vi "DecodeVireoToBotSpeak.vi"(3 "Via file":string="// Autogenerated Vireo assembly file\n// Generated on Fri Mar 27 10:48:11 2015\n\ndefine (c0 dv(.UInt32 1) )\ndefine (c1 dv(.UInt32 1) )\ndefine (c2 dv(c(\n    e(.String n0)   // Address\n    e(.String n1)   // Reply EOF\n    e(.String n2)   // Hardware\n    e(.Int8 n3)   // Retries\n    e(.Int32 n4)   // Timeout\n    e(.Boolean n5)   // Open?\n) ('' '' '' 0 0 false )) )\ndefine (c3 dv(.String '') )\n//---------------------------------------------------\n//VI Definition: BotSpeak_DIOWrite.vi\ndefine (videf1 dv(.VirtualInstrument (\n    c(\n        i(dv(.UInt32 1) local2)   // State\n        o(dv(.String '') local5)   // response\n        i(dv(c(\n            e(.String n0)   // Address\n            e(.String n1)   // Reply EOF\n            e(.String n2)   // Hardware\n            e(.Int8 n3)   // Retries\n            e(.Int32 n4)   // Timeout\n            e(.Boolean n5)   // Open?\n        ) ('' '' '' 0 0 false )) local1)   // Bot Settings\n        i(dv(.UInt32 0) local3)   // DIO Line\n        o(dv(c(\n            e(.String n0)   // Address\n            e(.String n1)   // Reply EOF\n            e(.String n2)   // Hardware\n            e(.Int8 n3)   // Retries\n            e(.Int32 n4)   // Timeout\n            e(.Boolean n5)   // Open?\n        ) ('' '' '' 0 0 false )) local4)   // Bot Settings\n    )\n    c(\n    )\n        clump(1\n        Copy(c2 local4 )\n        Copy(c3 local5 )\n//--- end of vi\n    )\n)))\n//---------------------------------------------------\n//VI Definition: TestingVI.vi\ndefine (videf2 dv(.VirtualInstrument (\n    c(\n    )\n        clump(1\n        videf1(c0 * * c1 *)\n//--- end of vi\n    )\n)))\nenqueue (videf2)\n") -> (1 "BotSpeak":string="SET DIO[1],1\n")   [LabVIEW 2014]
panel:
  out "Array 3":string[](array[string])=["", "", "", "", "BotSpeak_DIOWrite.vi", "TestingVI.vi", ""]
  out "Params":cluster{"Constant":string, "value":string}[](array[cluster])=[{"Constant"="videf1", "value"="SET DIO[#],#: 3 0 \n"}, {"Constant"="c3", "value"="''"}, {"Constant"="c2", "value"="   e(.String n0)   // Address\n    e(.String n1)   // Reply EOF\n    e(.String n2)   // Hardware\n    e(.Int8 n3)   // Retries\n    e(.Int32 n4)   // Timeout\n    e(.Boolean n5)   // Open?\n) ('' '' '' 0 0 false )"}, {"Constant"="c1", "value"="1"}, {"Constant"="c0", "value"="1"}]
  out "Array":T1(array[cluster])=[{"command"="define", "Contents"="c0 dv(.UInt32 1)", "previous comment"="// Generated on Fri Mar 27 10:48:11 2015"}, {"command"="define", "Contents"="c1 dv(.UInt32 1)", "previous comment"=""}, {"command"="define", "Contents"="c2 dv(c(\n    e(.String n0)   // Address\n    e(.String n1)   // Reply EOF\n    e(.String n2)   // Hardware\n    e(.Int8 n3)   // Retries\n    e(.Int32 n4)   // Timeout\n    e(.Boolean n5)   // Open?\n) ('' '' '' 0 0 false ))", "previous comment"=""}, {"command"="define", "Contents"="c3 dv(.String '')", "previous comment"=""}, {"command"="define", "Contents"="videf1 dv(.VirtualInstrument (\n    c(\n        i(dv(.UInt32 1) local2)   // State\n        o(dv(.String '') local5)   // response\n        i(dv(c(\n            e(.String n0)   // Address\n            e(.String n1)   // Reply EOF\n            e(.String n2)   // Hardware\n            e(.Int8 n3)   // Retries\n            e(.Int32 n4)   // Timeout\n            e(.Boolean n5)   // Open?\n        ) ('' '' '' 0 0 false )) local1)   // Bot Settings\n        i(dv(.UInt32 0) local3)   // DIO Line\n        o(dv(c(\n            e(.String n0)   // Address\n            e(.String n1)   // Reply EOF\n            e(.String n2)   // Hardware\n            e(.Int8 n3)   // Retries\n            e(.Int32 n4)   // Timeout\n            e(.Boolean n5)   // Open?\n        ) ('' '' '' 0 0 false )) local4)   // Bot Settings\n    )\n    c(\n    )\n        clump(1\n        Copy(c2 local4 )\n        Copy(c3 local5 )\n//--- end of vi\n    )\n))", "previous comment"="//VI Definition: BotSpeak_DIOWrite.vi"}, {"command"="define", "Contents"="videf2 dv(.VirtualInstrument (\n    c(\n    )\n        clump(1\n        videf1(c0 * * c1 *)\n//--- end of vi\n    )\n))", "previous comment"="//VI Definition: TestingVI.vi"}, {"command"="enqueue", "Contents"="videf2", "previous comment"=""}]
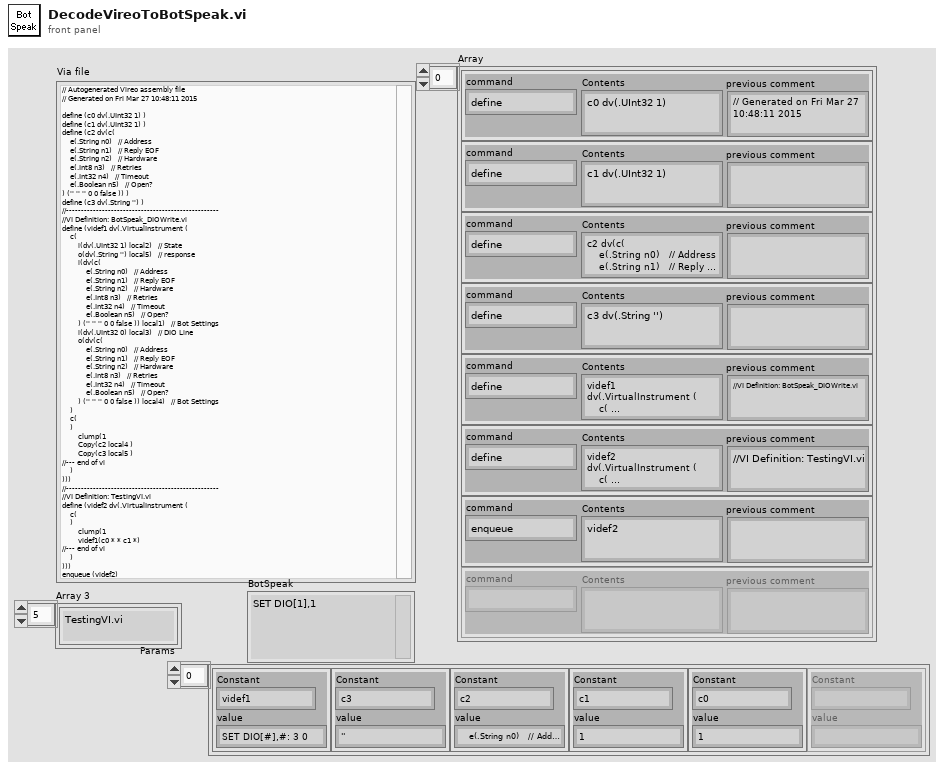
[diagram p1: front panel]
types:
  T1 = cluster{"command":string, "Contents":string, "previous comment":string}[]
  T2 = cluster{"Contents":string, "Contents 2":string}[]
  T3 = cluster{"command":string, "Contents":string, "Via file":string}
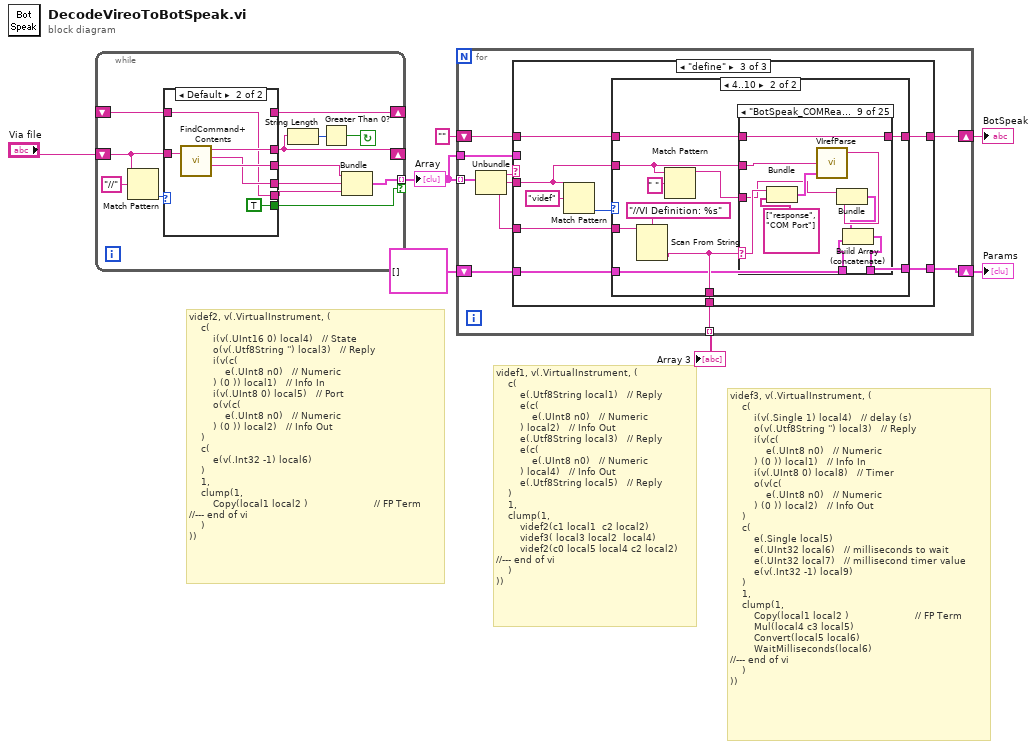
[diagram p0: block diagram]
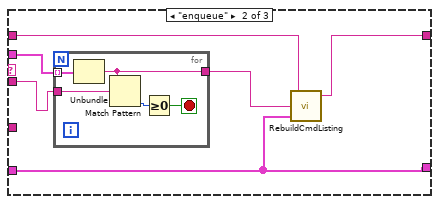
[diagram p3: hidden frame]
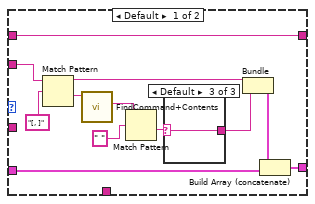
[diagram p4: hidden frame]
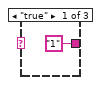
[diagram p5: hidden frame]
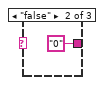
[diagram p6: hidden frame]
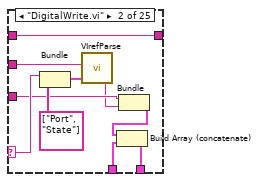
[diagram p8: hidden frame]
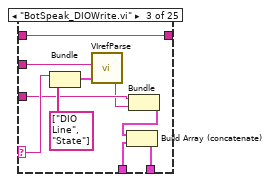
[diagram p9: hidden frame]
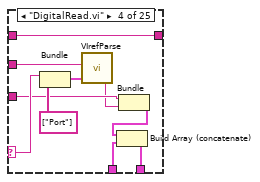
[diagram p10: hidden frame]
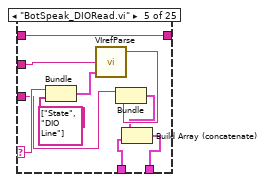
[diagram p11: hidden frame]
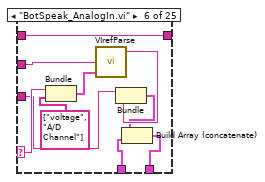
[diagram p12: hidden frame]
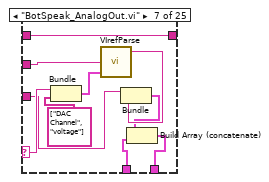
[diagram p13: hidden frame]
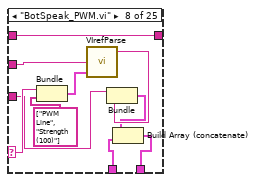
[diagram p14: hidden frame]
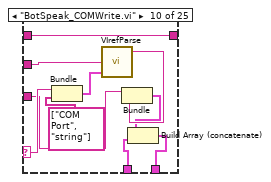
[diagram p15: hidden frame]
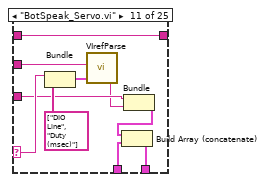
[diagram p16: hidden frame]
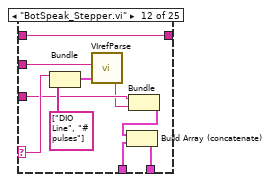
[diagram p17: hidden frame]
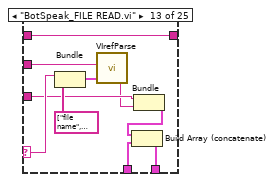
[diagram p18: hidden frame]
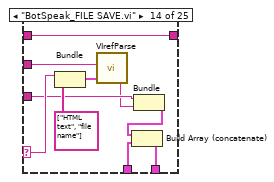
[diagram p19: hidden frame]
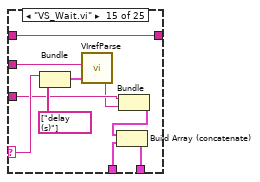
[diagram p20: hidden frame]
diagram:
  # "videf3, v(.VirtualInstrument, (\n    c(\n        i(v(.Single 1) local4)   // delay (s)\n        o(v(.Utf8String '') local3)   // Reply\n        i(v(c(\n            e(.UInt8 n0)   // Numeric\n        ) (0 )) local1)   // Info In\n        i(v(.UInt8 0) local8)   // Timer\n        o(v(c(\n            e(.UInt8 n0)   // Numeric\n        ) (0 )) local2)   // Info Out\n    )\n    c(\n        e(.Single local5)\n        e(.UInt32 local6)   // milliseconds to wait\n        e(.UInt32 local7)   // millisecond timer value\n        e(v(.Int32 -1) local9)\n    )\n    1,\n    clump(1,\n        Copy(local1 local2 )                      // FP Term\n        Mul(local4 c3 local5)\n        Convert(local5 local6)\n        WaitMilliseconds(local6)\n//--- end of vi\n    )\n))"
  # "videf1, v(.VirtualInstrument, (\n    c(\n        e(.Utf8String local1)   // Reply\n        e(c(\n            e(.UInt8 n0)   // Numeric\n        ) local2)   // Info Out\n        e(.Utf8String local3)   // Reply\n        e(c(\n            e(.UInt8 n0)   // Numeric\n        ) local4)   // Info Out\n        e(.Utf8String local5)   // Reply\n    )\n    1,\n    clump(1,\n        videf2(c1 local1  c2 local2)\n        videf3( local3 local2  local4)\n        videf2(c0 local5 local4 c2 local2)\n//--- end of vi\n    )\n))"
  # "videf2, v(.VirtualInstrument, (\n    c(\n        i(v(.UInt16 0) local4)   // State\n        o(v(.Utf8String '') local3)   // Reply\n        i(v(c(\n            e(.UInt8 n0)   // Numeric\n        ) (0 )) local1)   // Info In\n        i(v(.UInt8 0) local5)   // Port\n        o(v(c(\n            e(.UInt8 n0)   // Numeric\n        ) (0 )) local2)   // Info Out\n    )\n    c(\n        e(v(.Int32 -1) local6)\n    )\n    1,\n    clump(1,\n        Copy(local1 local2 )                      // FP Term\n//--- end of vi\n    )\n))"
  n1 = while {
    shift-right: [w20] -> _
    shift-left: "Via file" -> [w14]
    tunnel: [w15] -> w1 mode=indexing if=w9
    shift-right: [w11] -> _
    shift-left: _ -> [w10]
    stop <- w18 continue-if-true
    n2 = Match Pattern(string=w14, regular expression="//") -> (offset past match=w12:i32)  [unwired: 1 in, 3 out]
    n3 = case shown="Default" w12 {
      tunnel: [w23 w31] -> w20
      tunnel: ["//" ("regular expression") w30] -> w17
      tunnel: [w21 w29] -> w16
      tunnel: w14 -> [w25 w28]
      tunnel: [w21 _] -> w11
      tunnel: [_ w27] -> w8
      tunnel: w10 -> [_ w27]
      tunnel: [_ TRUE] -> w9
      frame 0..2 {
        n4 = Match Pattern(string=w25, regular expression="\n") -> (before substring=w21:string, after substring=w23:string)  [unwired: 1 in, 2 out]
      }
      frame Default {
        n5 = call <vilib>:"FindCommand+Contents.vi"("Via file in"=w28) -> ("left"=w31:string, "Contents"=w29:string, "command"=w30:string)  [unwired: 1 in, 1 out]
      }
    }
    n6 = String Length(string=w20) -> (length=w19:i32)
    n7 = Greater Than 0?(x=w19) -> (x > 0?=w18:bool)
    n8 = Bundle("command"=w17, "Contents"=w16, "Via file"=w8) -> (w15:T3)  [unwired: 1 in]
  }
  "Array" <- w1
  n9 = for {
    tunnel: w1 -> [w41] mode=indexing
    shift-right: [w36] -> w5
    shift-left: "" -> [w37]
    shift-right: [w35] -> w3
    shift-left: T2 [] -> [w34]
    tunnel: [w33] -> w2 mode=indexing
    tunnel: w1 -> [w32]
    n10 = Unbundle(w41) -> ("command"=w40:string, "Contents"=w39:string, "Via file"=w38:string)
    n11 = case shown="\"define\"" w40 {
      tunnel: w39 -> [_ w46 w58]
      tunnel: w38 -> [_ _ w61]
      tunnel: w37 -> [w42 w48 w60]
      tunnel: [w42 w49 w59] -> w36
      tunnel: [w43 w44 w57] -> w35
      tunnel: w34 -> [w43 w44 w56]
      tunnel: [_ _ w55] -> w33
      tunnel: w32 -> [_ w47 _]
      frame Default {
      }
      frame "enqueue" {
        n12 = for {
          tunnel: w47 -> [w54] mode=indexing
          tunnel: w46 -> [w53]
          tunnel: [w50] -> w45
          stop <- w51 stop-if-true
          n13 = Unbundle(w54) -> ("Contents"=w50:string)  [unwired: 2 out]
          n14 = Match Pattern(string=w50, regular expression=w53) -> (offset past match=w52:i32)  [unwired: 1 in, 3 out]
          n15 = Greater Or Equal To 0?(x=w52) -> (x >= 0?=w51:bool)
        }
        n16 = call <vilib>:"RebuildCmdListing.vi"("Params"=w44, "Contents"=w45, "String in"=w48) -> ("String out"=w49:string)  [unwired: 1 in, 1 out]
      }
      frame "define" {
        n17 = Match Pattern(string=w58, regular expression="videf") -> (offset past match=w62:i32)  [unwired: 1 in, 3 out]
        n18 = case shown="4..10" w62 {
          tunnel: w61 -> [_ w88]
          tunnel: w60 -> [w75 w86]
          tunnel: [w75 w85] -> w59
          tunnel: w58 -> [w73 w83]
          tunnel: [w67 w79] -> w57
          tunnel: w56 -> [w66 w80]
          tunnel: [_ w84] -> w55
          frame Default {
            n19 = Match Pattern(string=w73, regular expression="[, ]") -> (before substring=w71:string, after substring=w72:string)  [unwired: 1 in, 2 out]
            n20 = call <vilib>:"FindCommand+Contents.vi"("Via file in"=w72) -> ("Contents"=w70:string)  [unwired: 1 in, 3 out]
            n21 = Match Pattern(string=w70, regular expression=" ") -> (after substring=w65:string)  [unwired: 1 in, 3 out]
            n22 = case shown="Default" w65 {
              selector: w65 -> [_ _ w78]
              tunnel: ["1" "0" w78] -> w64
              frame "true" {
              }
              frame "false" {
              }
              frame Default {
              }
            }
            n23 = Bundle("Contents"=w71, w64) -> (w68:cluster{"Contents":string, string})  [unwired: 1 in]
            n24 = Build Array (concatenate)(w68, w66) -> (w67:T2)
          }
          frame 4..10 {
            n25 = Scan From String(format string="//VI Definition: %s" ("regular expression"), input string=w88) -> (output 1=w84:string)  [unwired: 3 in, 3 out]
            n26 = Match Pattern(string=w83, regular expression=" ") -> (before substring=w81:string)  [unwired: 1 in, 3 out]
            n27 = case shown="\"BotSpeak_COMRead.vi\"" w84 {
              selector: w84 -> [_ w99 w109 w119 w128 w137 w147 w157 w167 w177 w189 w199 w209 w219 w229 w239 w249 _ _ _ _ w267 w277 w287 w297]
              tunnel: w86 -> [w90 w96 w106 w116 w130 w140 w150 w160 w170 w180 w186 w196 w206 w216 w226 w236 w246 w252 w254 w256 w258 w264 w274 w284 w294]
              tunnel: [w90 w96 w106 w116 w130 w140 w150 w160 w170 w180 w186 w196 w206 w216 w226 w236 w246 w252 w254 w256 w258 w264 w274 w284 w294] -> w85
              tunnel: w83 -> [_ w100 w110 w120 w129 w139 w149 w159 w169 w179 w190 w200 w210 w220 w230 w240 w250 _ _ _ _ w268 w278 w288 w298]
              tunnel: w81 -> [_ w95 w105 w115 w126 w134 w145 w155 w165 w175 w185 w195 w205 w215 w225 w235 w245 _ _ _ _ w263 w273 w283 w293]
              tunnel: w80 -> [w89 w92 w102 w112 w124 w132 w143 w153 w163 w173 w182 w192 w202 w212 w222 w232 w242 w251 w253 w255 w257 w260 w270 w280 w290]
              tunnel: [w89 w91 w101 w111 w123 w131 w142 w152 w162 w172 w181 w191 w201 w211 w221 w231 w241 w251 w253 w255 w257 w259 w269 w279 w289] -> w79
              frame Default {
              }
              frame "DigitalWrite.vi" {
                n28 = Bundle(w99, string[] ["Port", "State"]) -> (w97:cluster{string, string[]})  [unwired: 1 in]
                n29 = call <vilib>:"VIrefParse.vi"("Params"=w97, "VIA"=w100) -> ("String out"=w94:string)  [unwired: 3 in]
                n30 = Bundle("Contents"=w95, "String out"=w94) -> (w93:cluster{"Contents":string, "String out":string})  [unwired: 1 in]
                n31 = Build Array (concatenate)(w93, w92) -> (w91:T2)
              }
              frame "BotSpeak_DIOWrite.vi" {
                n32 = Bundle(w109, string[] ["DIO Line", "State"]) -> (w107:cluster{string, string[]})  [unwired: 1 in]
                n33 = call <vilib>:"VIrefParse.vi"("Params"=w107, "VIA"=w110) -> ("String out"=w104:string)  [unwired: 3 in]
                n34 = Bundle("Contents"=w105, "String out"=w104) -> (w103:cluster{"Contents":string, "String out":string})  [unwired: 1 in]
                n35 = Build Array (concatenate)(w103, w102) -> (w101:T2)
              }
              frame "DigitalRead.vi" {
                n36 = Bundle(w119, string[] ["Port"]) -> (w117:cluster{string, string[]})  [unwired: 1 in]
                n37 = call <vilib>:"VIrefParse.vi"("Params"=w117, "VIA"=w120) -> ("String out"=w114:string)  [unwired: 3 in]
                n38 = Bundle("Contents"=w115, "String out"=w114) -> (w113:cluster{"Contents":string, "String out":string})  [unwired: 1 in]
                n39 = Build Array (concatenate)(w113, w112) -> (w111:T2)
              }
              frame "BotSpeak_DIORead.vi" {
                n40 = Bundle(w128, string[] ["State", "DIO Line"]) -> (w121:cluster{string, string[]})  [unwired: 1 in]
                n41 = call <vilib>:"VIrefParse.vi"("Params"=w121, "VIA"=w129) -> ("String out"=w127:string)  [unwired: 3 in]
                n42 = Bundle("Contents"=w126, "String out"=w127) -> (w125:cluster{"Contents":string, "String out":string})  [unwired: 1 in]
                n43 = Build Array (concatenate)(w125, w124) -> (w123:T2)
              }
              frame "BotSpeak_AnalogIn.vi" {
                n44 = Bundle(w137, string[] ["voltage", "A/D Channel"]) -> (w138:cluster{string, string[]})  [unwired: 1 in]
                n45 = call <vilib>:"VIrefParse.vi"("Params"=w138, "VIA"=w139) -> ("String out"=w135:string)  [unwired: 3 in]
                n46 = Bundle("Contents"=w134, "String out"=w135) -> (w133:cluster{"Contents":string, "String out":string})  [unwired: 1 in]
                n47 = Build Array (concatenate)(w133, w132) -> (w131:T2)
              }
              frame "BotSpeak_AnalogOut.vi" {
                n48 = Bundle(w147, string[] ["DAC Channel", "voltage"]) -> (w148:cluster{string, string[]})  [unwired: 1 in]
                n49 = call <vilib>:"VIrefParse.vi"("Params"=w148, "VIA"=w149) -> ("String out"=w146:string)  [unwired: 3 in]
                n50 = Bundle("Contents"=w145, "String out"=w146) -> (w144:cluster{"Contents":string, "String out":string})  [unwired: 1 in]
                n51 = Build Array (concatenate)(w144, w143) -> (w142:T2)
              }
              frame "BotSpeak_PWM.vi" {
                n52 = Bundle(w157, string[] ["PWM Line", "Strength (100)"]) -> (w158:cluster{string, string[]})  [unwired: 1 in]
                n53 = call <vilib>:"VIrefParse.vi"("Params"=w158, "VIA"=w159) -> ("String out"=w156:string)  [unwired: 3 in]
                n54 = Bundle("Contents"=w155, "String out"=w156) -> (w154:cluster{"Contents":string, "String out":string})  [unwired: 1 in]
                n55 = Build Array (concatenate)(w154, w153) -> (w152:T2)
              }
              frame "BotSpeak_COMRead.vi" {
                n56 = Bundle(w167, string[] ["response", "COM Port"]) -> (w168:cluster{string, string[]})  [unwired: 1 in]
                n57 = call <vilib>:"VIrefParse.vi"("Params"=w168, "VIA"=w169) -> ("String out"=w166:string)  [unwired: 3 in]
                n58 = Bundle("Contents"=w165, "String out"=w166) -> (w164:cluster{"Contents":string, "String out":string})  [unwired: 1 in]
                n59 = Build Array (concatenate)(w164, w163) -> (w162:T2)
              }
              frame "BotSpeak_COMWrite.vi" {
                n60 = Bundle(w177, string[] ["COM Port", "string"]) -> (w178:cluster{string, string[]})  [unwired: 1 in]
                n61 = call <vilib>:"VIrefParse.vi"("Params"=w178, "VIA"=w179) -> ("String out"=w176:string)  [unwired: 3 in]
                n62 = Bundle("Contents"=w175, "String out"=w176) -> (w174:cluster{"Contents":string, "String out":string})  [unwired: 1 in]
                n63 = Build Array (concatenate)(w174, w173) -> (w172:T2)
              }
              frame "BotSpeak_Servo.vi" {
                n64 = Bundle(w189, string[] ["DIO Line", "Duty (msec)"]) -> (w187:cluster{string, string[]})  [unwired: 1 in]
                n65 = call <vilib>:"VIrefParse.vi"("Params"=w187, "VIA"=w190) -> ("String out"=w184:string)  [unwired: 3 in]
                n66 = Bundle("Contents"=w185, "String out"=w184) -> (w183:cluster{"Contents":string, "String out":string})  [unwired: 1 in]
                n67 = Build Array (concatenate)(w183, w182) -> (w181:T2)
              }
              frame "BotSpeak_Stepper.vi" {
                n68 = Bundle(w199, string[] ["DIO Line", "# pulses"]) -> (w197:cluster{string, string[]})  [unwired: 1 in]
                n69 = call <vilib>:"VIrefParse.vi"("Params"=w197, "VIA"=w200) -> ("String out"=w194:string)  [unwired: 3 in]
                n70 = Bundle("Contents"=w195, "String out"=w194) -> (w193:cluster{"Contents":string, "String out":string})  [unwired: 1 in]
                n71 = Build Array (concatenate)(w193, w192) -> (w191:T2)
              }
              frame "BotSpeak_FILE READ.vi" {
                n72 = Bundle(w209, string[] ["file name", "DIO Line"]) -> (w207:cluster{string, string[]})  [unwired: 1 in]
                n73 = call <vilib>:"VIrefParse.vi"("Params"=w207, "VIA"=w210) -> ("String out"=w204:string)  [unwired: 3 in]
                n74 = Bundle("Contents"=w205, "String out"=w204) -> (w203:cluster{"Contents":string, "String out":string})  [unwired: 1 in]
                n75 = Build Array (concatenate)(w203, w202) -> (w201:T2)
              }
              frame "BotSpeak_FILE SAVE.vi" {
                n76 = Bundle(w219, string[] ["HTML text", "file name"]) -> (w217:cluster{string, string[]})  [unwired: 1 in]
                n77 = call <vilib>:"VIrefParse.vi"("Params"=w217, "VIA"=w220) -> ("String out"=w214:string)  [unwired: 3 in]
                n78 = Bundle("Contents"=w215, "String out"=w214) -> (w213:cluster{"Contents":string, "String out":string})  [unwired: 1 in]
                n79 = Build Array (concatenate)(w213, w212) -> (w211:T2)
              }
              frame "VS_Wait.vi" {
                n80 = Bundle(w229, string[] ["delay (s)"]) -> (w227:cluster{string, string[]})  [unwired: 1 in]
                n81 = call <vilib>:"VIrefParse.vi"("Params"=w227, "VIA"=w230) -> ("String out"=w224:string)  [unwired: 3 in]
                n82 = Bundle("Contents"=w225, "String out"=w224) -> (w223:cluster{"Contents":string, "String out":string})  [unwired: 1 in]
                n83 = Build Array (concatenate)(w223, w222) -> (w221:T2)
              }
              frame "BotSpeak_Wait.vi" {
                n84 = Bundle(w239, string[] ["Wait (sec)"]) -> (w237:cluster{string, string[]})  [unwired: 1 in]
                n85 = call <vilib>:"VIrefParse.vi"("Params"=w237, "VIA"=w240) -> ("String out"=w234:string)  [unwired: 3 in]
                n86 = Bundle("Contents"=w235, "String out"=w234) -> (w233:cluster{"Contents":string, "String out":string})  [unwired: 1 in]
                n87 = Build Array (concatenate)(w233, w232) -> (w231:T2)
              }
              frame "BotSpeak_Waitms.vi" {
                n88 = Bundle(w249, string[] ["Wait (ms)"]) -> (w247:cluster{string, string[]})  [unwired: 1 in]
                n89 = call <vilib>:"VIrefParse.vi"("Params"=w247, "VIA"=w250) -> ("String out"=w244:string)  [unwired: 3 in]
                n90 = Bundle("Contents"=w245, "String out"=w244) -> (w243:cluster{"Contents":string, "String out":string})  [unwired: 1 in]
                n91 = Build Array (concatenate)(w243, w242) -> (w241:T2)
              }
              frame "BotSpeak_LoadScript.vi" {
              }
              frame "BotSpeak_RunScript.vi" {
              }
              frame "BotSpeak_RunWaitScript.vi" {
              }
              frame "BotSpeak_DebugScript.vi" {
              }
              frame "BotSpeak_GetVar.vi" {
                n92 = Bundle(w267, string[] ["value", "Variable In"]) -> (w265:cluster{string, string[]})  [unwired: 1 in]
                n93 = call <vilib>:"VIrefParse.vi"("Params"=w265, "VIA"=w268) -> ("String out"=w262:string)  [unwired: 3 in]
                n94 = Bundle("Contents"=w263, "String out"=w262) -> (w261:cluster{"Contents":string, "String out":string})  [unwired: 1 in]
                n95 = Build Array (concatenate)(w261, w260) -> (w259:T2)
              }
              frame "BotSpeak_Set.vi" {
                n96 = Bundle(w277, string[] ["Variable In", "value"]) -> (w275:cluster{string, string[]})  [unwired: 1 in]
                n97 = call <vilib>:"VIrefParse.vi"("Params"=w275, "VIA"=w278) -> ("String out"=w272:string)  [unwired: 3 in]
                n98 = Bundle("Contents"=w273, "String out"=w272) -> (w271:cluster{"Contents":string, "String out":string})  [unwired: 1 in]
                n99 = Build Array (concatenate)(w271, w270) -> (w269:T2)
              }
              frame "BotSpeak_GetVer.vi" {
                n100 = Bundle(w287, string[] ["version"]) -> (w285:cluster{string, string[]})  [unwired: 1 in]
                n101 = call <vilib>:"VIrefParse.vi"("Params"=w285, "VIA"=w288) -> ("String out"=w282:string)  [unwired: 3 in]
                n102 = Bundle("Contents"=w283, "String out"=w282) -> (w281:cluster{"Contents":string, "String out":string})  [unwired: 1 in]
                n103 = Build Array (concatenate)(w281, w280) -> (w279:T2)
              }
              frame "BotSpeak_System.vi" {
                n104 = Bundle(w297, string[] ["Variable In", "Values sent"]) -> (w295:cluster{string, string[]})  [unwired: 1 in]
                n105 = call <vilib>:"VIrefParse.vi"("Params"=w295, "VIA"=w298) -> ("String out"=w292:string)  [unwired: 3 in]
                n106 = Bundle("Contents"=w293, "String out"=w292) -> (w291:cluster{"Contents":string, "String out":string})  [unwired: 1 in]
                n107 = Build Array (concatenate)(w291, w290) -> (w289:T2)
              }
            }
          }
        }
      }
    }
  }
  "BotSpeak" <- w5
  "Params" <- w3
  "Array 3" <- w2
